vi "git_options_dialog.vi"(11 "Working Dir":path) -> ()   [LabVIEW 2020, in "AJ_QuickDrop_Git.lvlib"]
uses:
  <resource>/dialog/QuickDrop/plugins/AJ_QD_Git/AJ_QuickDrop_Git.lvlib
panel:
  in  "Select":bool
  in  "Git Option":i32(listbox)
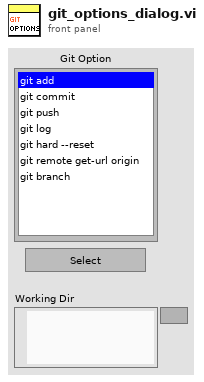
[diagram p1: front panel]
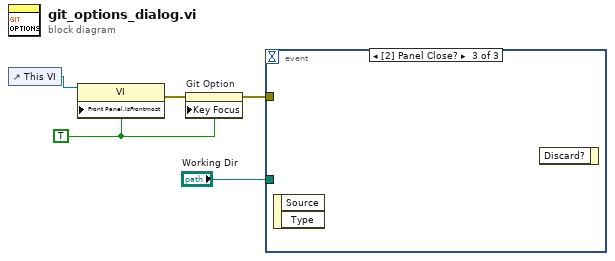
[diagram p0: block diagram]
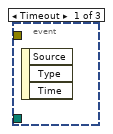
[diagram p2: hidden frame]
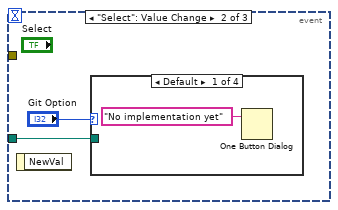
[diagram p3: hidden frame]
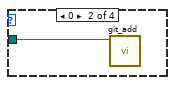
[diagram p4: hidden frame]
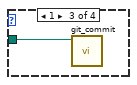
[diagram p5: hidden frame]
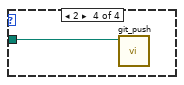
[diagram p6: hidden frame]
diagram:
  w3 = TRUE ("Front Panel Window:Is Frontmost")
  n1 = control-ref of="This VI"() -> (w4:refnum<vi>)
  n2 = property class="VI"(reference=w4, "Front Panel.IsFrontmost"=w3) -> (error out=w2:errorcluster)  [unwired: 1 in, 1 out]
  n3 = property on="Git Option" class="LstBox (strict)"(error in=w2, "Key Focus"=w3) -> (error out=w1:errorcluster)  [unwired: 1 in, 1 out]
  n4 = event shown="[2] Panel Close?" {
    selector: _ -> [_ _ _]
    dyn-events: _ -> [_ _ _]
    timeout: _ -> [_ _ _]
    tunnel: "Working Dir" -> [_ w6 _]
    tunnel: w1 -> [_ _ _]
    event Timeout {
      n5 = event-data() -> ()  [unwired: 1 in, 3 out]
    }
    event "Select": Value Change {
      n6 = event-data() -> ()  [unwired: 1 in, 1 out]
      n7 = case shown="Default" "Git Option" {
        tunnel: w6 -> [_ w9 w10 w11]
        frame Default {
          n8 = One Button Dialog(message="No implementation yet") -> ()  [unwired: 1 in, 1 out]
        }
        frame 0 {
          n9 = call <resource>:"git_add.vi"("Working Dir"=w9) -> ()  [unwired: 11 in]
        }
        frame 1 {
          n10 = call <resource>:"git_commit.vi"("Working Dir"=w10) -> ()  [unwired: 11 in]
        }
        frame 2 {
          n11 = call <resource>:"git_push.vi"("Working Dir"=w11) -> ()  [unwired: 11 in]
        }
      }
    }
    event Panel Close? {
      n12 = event-data() -> ()  [unwired: 1 in, 2 out]
      n13 = event-data() -> ()  [unwired: 2 in, 1 out]
    }
  }
